vi "SSI_Save.vi"(0 "file path (dialog if empty)":path caption="Save path", 1 "1D data":dbl[](array[numeric]), 2 "2D data":dbl[][](array[numeric]), 3 "Instrument Mode":T1(ring), 4 "Save Button":bool) -> ()   [LabVIEW 2011]
uses:
  <vilib>/Utility/file.llb/Write To Spreadsheet File (string).vi
  <vilib>/Utility/file.llb/Write To Spreadsheet File (DBL).vi
panel:
  out "Index_flag":i32
  out "Sample_array":dbl[][](array[numeric])
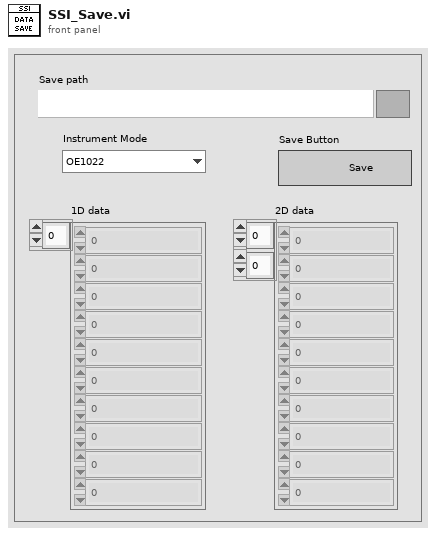
[diagram p1: front panel]
types:
  T1 = enum16{"OE1022", "OE1022D", "OE1201", "OE2031&OE2041", "OE1311&OE1351", "OE2052"}
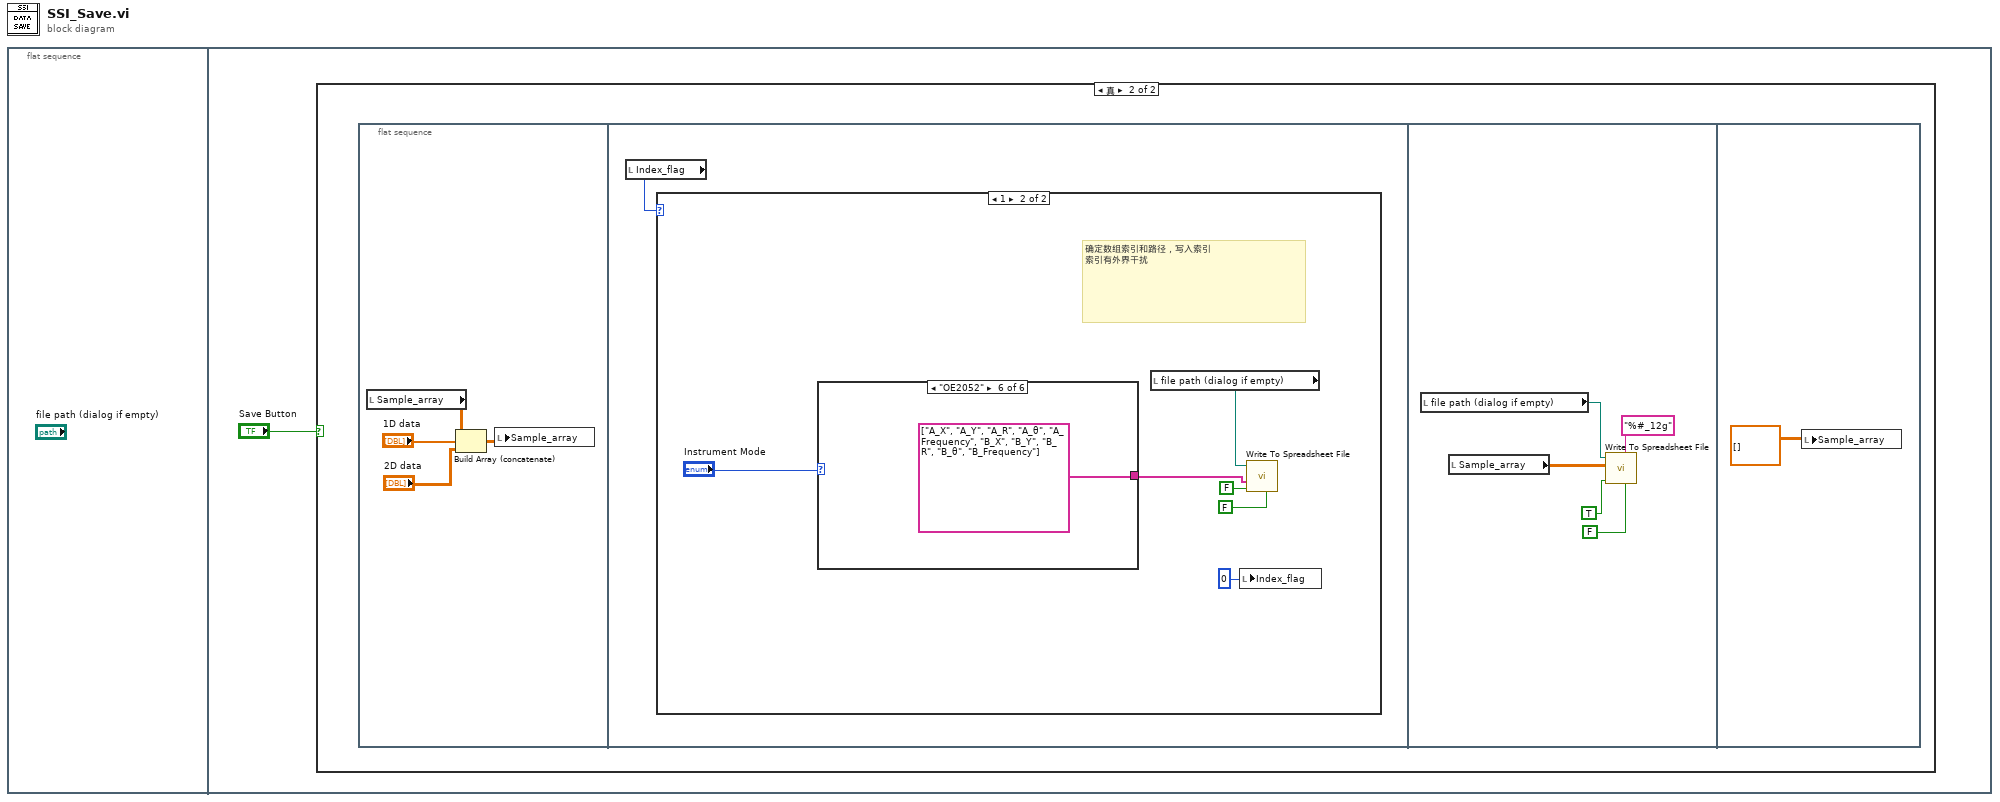
[diagram p0: block diagram]
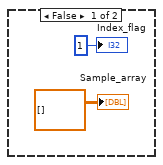
[diagram p2: hidden frame]
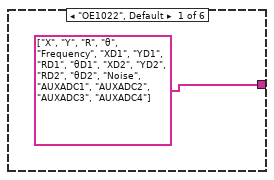
[diagram p4: hidden frame]
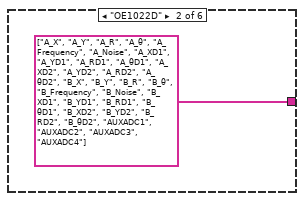
[diagram p5: hidden frame]
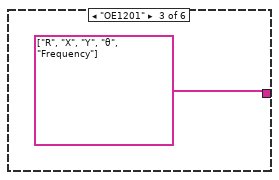
[diagram p6: hidden frame]
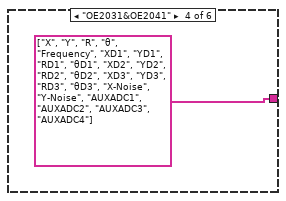
[diagram p7: hidden frame]
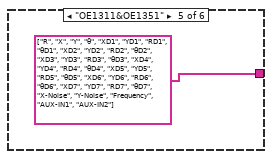
[diagram p8: hidden frame]
diagram:
  n1 = flat-sequence {
    frame #0 {
    }
    frame #1 {
      n2 = case shown="真" "Save Button" {
        frame False {
          "Index_flag" <- 1 ("Index_flag")
          "Sample_array" <- dbl[][] []
        }
        frame True {
          n3 = flat-sequence {
            frame #0 {
              n4 = local read "Sample_array"() -> (w5:dbl[][])
              n5 = Build Array (concatenate)(w5, "1D data", "2D data") -> (w7:dbl[][])
              n6 = local write "Sample_array"(w7) -> ()
            }
            frame #1 {
              n7 = local read "Index_flag"() -> (w8:i32)
              n8 = case shown="1" w8 {
                frame 0, Default {
                }
                frame 1 {
                  # "确定数组索引和路径，写入索引\n索引有外界干扰"
                  n9 = case shown="\"OE2052\"" "Instrument Mode" {
                    tunnel: [string[] ["X", "Y", "R", "θ", "Frequency", "XD1", "YD1", "RD1", "θD1", "XD2", "YD2", "RD2", "θD2", "Noise", "AUXADC1", "AUXADC2", "AUXADC3", "AUXADC4"] string[] ["A_X", "A_Y", "A_R", "A_θ", "A_Frequency", "A_Noise", "A_XD1", "A_YD1", "A_RD1", "A_θD1", "A_XD2", "A_YD2", "A_RD2", "A_θD2", "B_X", "B_Y", "B_R", "B_θ", "B_Frequency", "B_Noise", "B_XD1", "B_YD1", "B_RD1", "B_θD1", "B_XD2", "B_YD2", "B_RD2", "B_θD2", "AUXADC1", "AUXADC2", "AUXADC3", "AUXADC4"] ("输出数组") string[] ["R", "X", "Y", "θ", "Frequency"] string[] ["X", "Y", "R", "θ", "Frequency", "XD1", "YD1", "RD1", "θD1", "XD2", "YD2", "RD2", "θD2", "XD3", "YD3", "RD3", "θD3", "X-Noise", "Y-Noise", "AUXADC1", "AUXADC2", "AUXADC3", "AUXADC4"] string[] ["R", "X", "Y", "θ", "XD1", "YD1", "RD1", "θD1", "XD2", "YD2", "RD2", "θD2", "XD3", "YD3", "RD3", "θD3", "XD4", "YD4", "RD4", "θD4", "XD5", "YD5", "RD5", "θD5", "XD6", "YD6", "RD6", "θD6", "XD7", "YD7", "RD7", "θD7", "X-Noise", "Y-Noise", "Frequency", "AUX-IN1", "AUX-IN2"] string[] ["A_X", "A_Y", "A_R", "A_θ", "A_Frequency", "B_X", "B_Y", "B_R", "B_θ", "B_Frequency"]] -> w10
                    frame "OE1022", Default {
                    }
                    frame "OE1022D" {
                    }
                    frame "OE1201" {
                    }
                    frame "OE2031&OE2041" {
                    }
                    frame "OE1311&OE1351" {
                    }
                    frame "OE2052" {
                    }
                  }
                  n10 = local read "file path (dialog if empty)"() -> (w13:path)
                  n11 = local write "Index_flag"(0 ("Index_flag")) -> ()
                  n12 = call-poly <vilib>:"Write To Spreadsheet File.vi"("transpose? (no:F)"=FALSE, "append to file? (new file:F)"=FALSE, "1D data"=w10, "file path (dialog if empty)"=w13) -> ()  [unwired: 4 in, 1 out]
                }
              }
            }
            frame #2 {
              n13 = local read "file path (dialog if empty)"() -> (w24:path)
              n14 = local read "Sample_array"() -> (w25:dbl[][])
              n15 = call-poly <vilib>:"Write To Spreadsheet File.vi"("transpose? (no:F)"=FALSE, "format (%.3f)"="%#_12g", "append to file? (new file:F)"=TRUE, "2D data"=w25, "file path (dialog if empty)"=w24) -> ()  [unwired: 3 in, 1 out]
            }
            frame #3 {
              n16 = local write "Sample_array"(dbl[][] [] ("采样数组")) -> ()
            }
          }
        }
      }
    }
  }
